vi "Convert to Module Class.vi"(8 "error in":errorcluster, 10 "slot ref in":T1 format="%.0x", 11 "RSI Module in":refnum<class "RSI Module.lvclass">) -> (0 "error out":errorcluster, 2 "module":refnum<class "Module.lvclass">, 3 "RSI Module out":refnum<class "RSI Module.lvclass">)   [LabVIEW 2017, in "Modules.lvlib" / "RSI Module.lvclass"]
uses:
  RSI Module.lvclass
  niveristand-scan-engine-ethercat-custom-device/Custom Device Source/Scripting/Modules/Module/Module.lvclass
  <vilib>/NI Veristand/Custom Device API/Custom Device Item Ref.ctl
  Modules.lvlib
  <vilib>/NI Veristand/Custom Device API/Custom Device API.lvlib
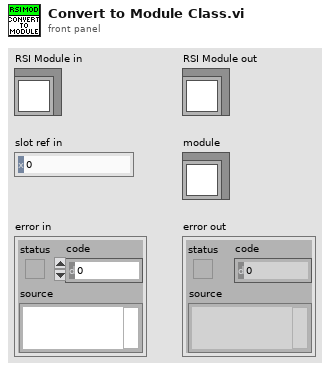
[diagram p1: front panel]
types:
  T1 = typedef "Custom Device API.lvlib/Custom Device Item Ref.ctl" = u64
  T2 = typedef "Modules.lvlib/RSI Module.lvclass/Module Models.ctl" = enum16{"Empty", "NI 9201", "NI 9203", "NI 9205", "NI 9206", "NI 9207", "NI 9208", "NI 9209", "NI 9210", "NI 9211", "NI 9212", "NI 9213", "NI 9214", "NI 9215", "NI 9216", "NI 9217", "NI 9219", "NI 9220", "NI 9221", "NI 9222", "NI 9223", "NI 9224", "NI 9225", "NI 9226", "NI 9227", "NI 9228", "NI 9229", "NI 9233", "NI 9234", "NI 9235", "NI 9236", "NI 9237", "NI 9239", "NI 9242", "NI 9244", "NI 9253", "NI 9263", "NI 9264", "NI 9265", "NI 9266", "NI 9269", "NI 9344", "NI 9350", "NI 9375", "NI 9401", "NI 9402", "NI 9403", "NI 9411", "NI 9421", "NI 9422", "NI 9423", "NI 9425", "NI 9426", "NI 9435", "NI 9436", "NI 9437", "NI 9472", "NI 9474", "NI 9475", "NI 9476", "NI 9477", "NI 9478", "NI 9481", "NI 9482", "NI 9485"}
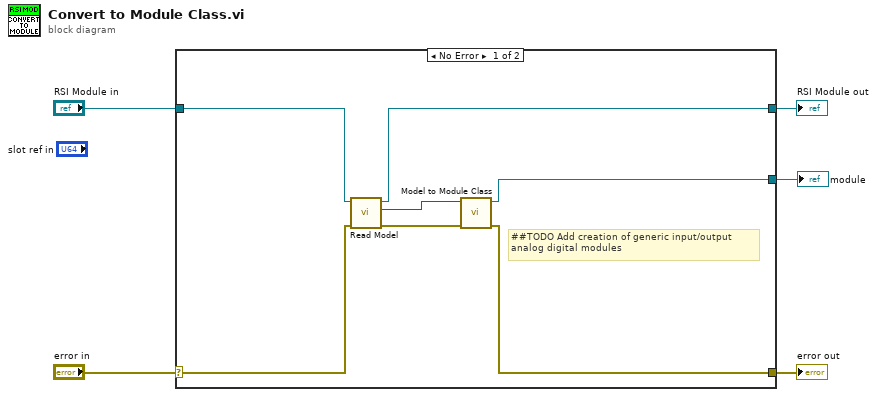
[diagram p0: block diagram]
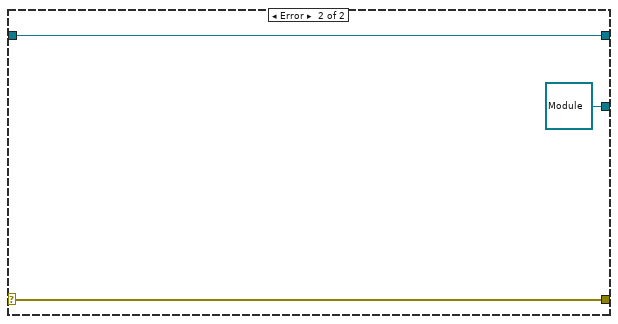
[diagram p2: hidden frame]
diagram:
  n1 = case shown="No Error" "error in" {
    selector: "error in" -> [w7 w15]
    tunnel: [w8 w15] -> w4
    tunnel: [w6 w14] -> w2
    tunnel: "RSI Module in" -> [w10 w14]
    tunnel: [w9 refnum<class "Module.lvclass"> refnum ("module")] -> w1
    frame No Error {
      # "##TODO Add creation of generic input/output\nanalog digital modules"
      n2 = call "Read Model.vi"("error in (no error)"=w7, "RSI Module in"=w10) -> ("error out"=w11:errorcluster, "Model"=w12:T2, "RSI Module out"=w6:refnum<class "RSI Module.lvclass">)  [unwired: 7 in]
      n3 = call "Model to Module Class.vi"("error in"=w11, "Module Model"=w12) -> ("error out"=w8:errorcluster, "module"=w9:refnum<class "Module.lvclass">)  [unwired: 8 in]
    }
    frame Error {
    }
  }
  "error out" <- w4
  "RSI Module out" <- w2
  "module" <- w1
